vi "Generate Time Data.vi"(3 "Time Offset":dbl, 4 "Sample Rate":dbl, 5 "Data":sgl[][](array[numeric])) -> (0 "Last Time":dbl, 2 "Array":sgl[][](array[numeric]))   [LabVIEW 2019]
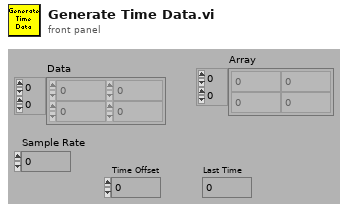
[diagram p1: front panel]
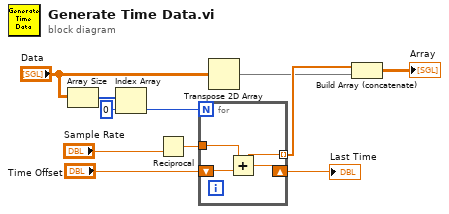
[diagram p0: block diagram]
diagram:
  n1 = Array Size(array="Data") -> (size(s)=w8:i32[])
  n2 = Index Array(array=w8, index=0) -> (element=w2:i32)
  n3 = Reciprocal(x="Sample Rate") -> (1/x=w3:dbl)
  n4 = for {
    N: w2 -> [_]
    tunnel: w3 -> [w13]
    shift-right: [w12] -> w6
    shift-left: "Time Offset" -> [w14]
    tunnel: [w12] -> w5 mode=indexing
    n5 = Add(x=w13, y=w14) -> (x+y=w12:dbl)
  }
  "Last Time" <- w6
  n6 = Transpose 2D Array(2D array="Data") -> (transposed array=w1:sgl[][])
  n7 = Build Array (concatenate)(w5, w1) -> (→"Array":dbl[][])
